vi "ScoreValidate.vi"(4 "Score":T2={"GUID"=0, "Score Mode Selector"=0, "Round Number"=0, "Full Score Entry"={"Elements"=[{"Name"="CO2 Balls Touching/Within Reservoir Model", "Value"="-1"}, {"Name"="Money Ball Touching/Within Reservoir Model", "Value"="-1"}, {"Name"="3+ Red/White Citizens in Pink Grid Area", "Value"="-1"}, {"Name"="# Upright Levee Blocks touching ONLY GREEN shores", "Value"="-1"}, {"Name"="# Upright Levee Blocks Touching any RED shore", "Value"="-1"}, {"Name"="Levee Test was Performed", "Value"="-1"}, {"Name"="Levee Test Wheel Blocked by NonLevee", "Value"="-1"}, {"Name"="Flood Barrier in Up Position", "Value"="-1"}, {"Name"="Both Yellow Arrows Aligned", "Value"="-1"}, {"Name"="Team Robot Touching Only Yellow Grid Area", "Value"="-1"}, {"Name"="Both Insulation Touching Green Grid Area", "Value"="-1"}, {"Name"="Bicycle Touching Green Grid Area", "Value"="-1"}, {"Name"="Computer Touching Green Grid Area", "Value"="-1"}, {"Name"="House in Up Position", "Value"="-1"}, {"Name"="House Window Showing Black", "Value"="-1"}, {"Name"="House Window All The Way Open", "Value"="-1"}, {"Name"="3+ Black/White Scientists Touching Research Area", "Value"="-1"}, {"Name"="Money Ball Touching/Within Research Area Model", "Value"="-1"}, {"Name"="Polar Bear Touching/Within Research Area Model", "Value"="-1"}, {"Name"="Polar Bear Orientation (Sleeping/Upright)", "Value"="-1"}, {"Name"="Ice Core Pulled From Its Hole", "Value"="-1"}, {"Name"="Ice Buoy Upright and Within/Touching Research Area Model", "Value"="-1"}, {"Name"="Drilling Machine Touching/Within Research Area Model", "Value"="-1"}, {"Name"="Drill Assembly Completely Vertical", "Value"="-1"}, {"Name"="Team Robot Touching/Within Research Area Model", "Value"="-1"}, {"Name"="3+ Blue/Gray Leaders Touching Green Mountain/City Area", "Value"="-1"}, {"Name"="Ice Core in Base Area", "Value"="-1"}, {"Name"="Snowmobile Touching/Within Research Area Model", "Value"="-1"}], "Score"=0.0}} {"Score Mode Selector" items=["Automatic", "Manual"]}, 5 "Scores":T1 {"Score"."Score Mode Selector" items=["Automatic", "Manual"]}) -> (0 "Errors":string, 1 "Index":i32, 2 "Scores Out":T1 {"Score"."Score Mode Selector" items=["Automatic", "Manual"]})   [LabVIEW 2013]
uses:
  Full Score Entry.ctl
  ScoreEntry.ctl
  ScoreList.ctl
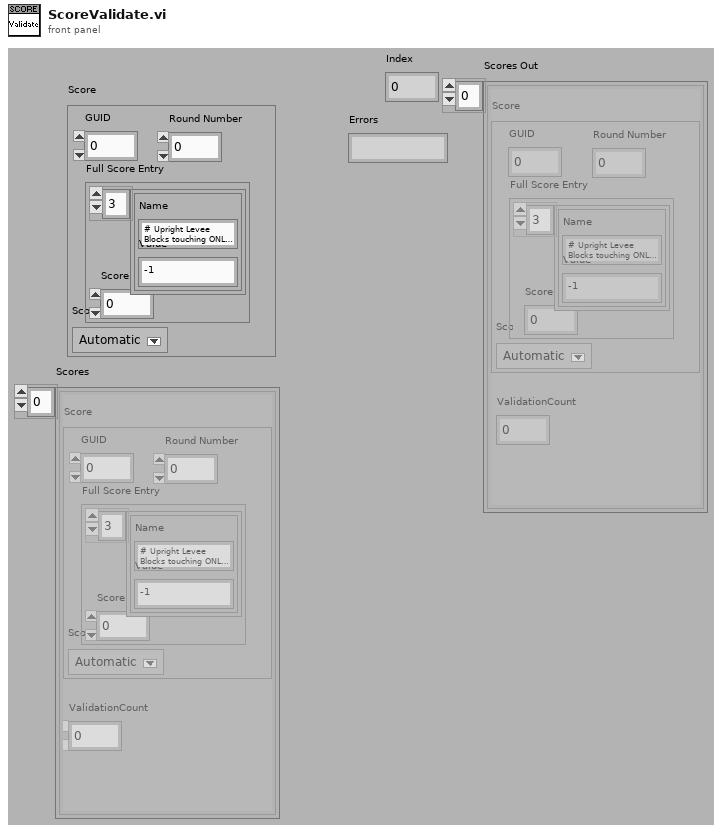
[diagram p1: front panel]
types:
  T1 = typedef "ScoreList.ctl" = cluster{"ValidationCount":u16, "Score":T2}[]
  T2 = typedef "Full Score Entry.ctl" = cluster{"GUID":u16, "Score Mode Selector":u16, "Round Number":u16, "Full Score Entry":T3}
  T3 = typedef "ScoreEntry.ctl" = cluster{"Elements":cluster{"Name":string, "Value":string}[], "Score":dbl}
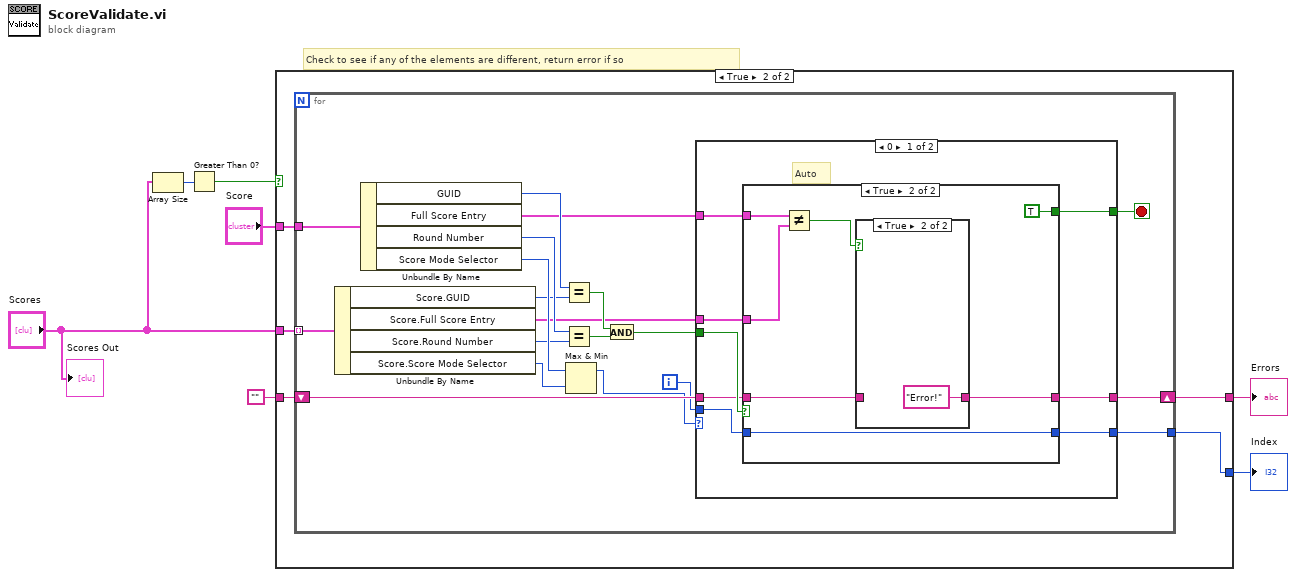
[diagram p0: block diagram]
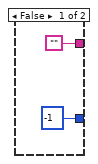
[diagram p2: hidden frame]
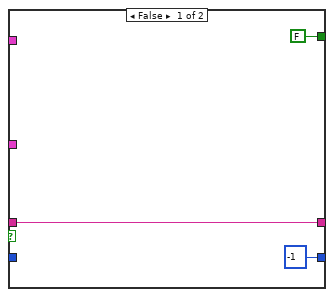
[diagram p3: hidden frame]
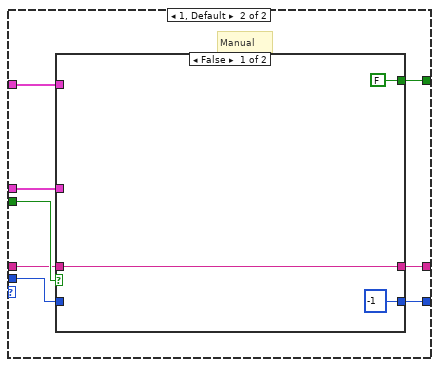
[diagram p5: hidden frame]
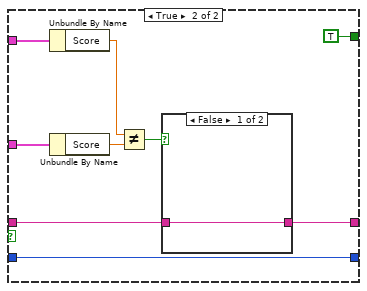
[diagram p6: hidden frame]
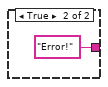
[diagram p7: hidden frame]
diagram:
  # "Check to see if any of the elements are different, return error if so"
  n1 = Array Size(array="Scores") -> (size(s)=w4:i32)
  n2 = Greater Than 0?(x=w4) -> (x > 0?=w3:bool)
  n3 = case shown="True" w3 {
    tunnel: "Score" -> [_ w14]
    tunnel: "" -> [_ w13]
    tunnel: ["" w12] -> w6
    tunnel: [-1 w11] -> w5
    tunnel: "Scores" -> [_ w10]
    frame False {
    }
    frame True {
      n4 = for {
        tunnel: w14 -> [w33]
        tunnel: w10 -> [w19] mode=indexing
        shift-right: [w25] -> w12
        shift-left: w13 -> [w26]
        tunnel: [w21] -> w11
        i -> [w22]
        stop <- w20 stop-if-true
        n5 = Unbundle By Name(w19) -> ("Score.GUID"=w18:u16, "Score.Full Score Entry"=w17:T3, "Score.Round Number"=w16:u16, "Score.Score Mode Selector"=w15:u16)
        n6 = Unbundle By Name(w33) -> ("GUID"=w32:u16, "Full Score Entry"=w27:T3, "Round Number"=w31:u16, "Score Mode Selector"=w24:u16)
        n7 = Equal?(x=w32, y=w18) -> (x = y?=w29:bool)
        n8 = Equal?(x=w31, y=w16) -> (x = y?=w30:bool)
        n9 = Max & Min(x=w24, y=w15) -> (max(x,y)=w23:u16)  [unwired: 1 out]
        n10 = And(x=w29, y=w30) -> (x .and. y?=w28:bool)
        n11 = case shown="0" w23 {
          tunnel: w28 -> [w41 w61]
          tunnel: w27 -> [w40 w60]
          tunnel: w17 -> [w39 w59]
          tunnel: w26 -> [w38 w58]
          tunnel: [w37 w57] -> w25
          tunnel: w22 -> [w36 w56]
          tunnel: [w35 w55] -> w21
          tunnel: [w34 w54] -> w20
          frame 0 {
            # "Auto"
            n12 = case shown="True" w41 {
              tunnel: w40 -> [_ w50]
              tunnel: w39 -> [_ w51]
              tunnel: w38 -> [w44 w48]
              tunnel: [w44 w47] -> w37
              tunnel: w36 -> [_ w46]
              tunnel: [-1 w46] -> w35
              tunnel: [FALSE TRUE] -> w34
              frame False {
              }
              frame True {
                n13 = Not Equal?(x=w50, y=w51) -> (x != y?=w49:bool)
                n14 = case shown="True" w49 {
                  tunnel: w48 -> [w52 _]
                  tunnel: [w52 "Error!"] -> w47
                  frame False {
                  }
                  frame True {
                  }
                }
              }
            }
          }
          frame 1, Default {
            # "Manual"
            n15 = case shown="False" w61 {
              tunnel: w60 -> [_ w69]
              tunnel: w59 -> [_ w70]
              tunnel: w58 -> [w64 w72]
              tunnel: [w64 w71] -> w57
              tunnel: w56 -> [_ w66]
              tunnel: [-1 w66] -> w55
              tunnel: [FALSE TRUE] -> w54
              frame False {
              }
              frame True {
                n16 = Unbundle By Name(w69) -> ("Score"=w68:dbl)
                n17 = Unbundle By Name(w70) -> ("Score"=w67:dbl)
                n18 = Not Equal?(x=w68, y=w67) -> (x != y?=w73:bool)
                n19 = case shown="False" w73 {
                  tunnel: w72 -> [w74 _]
                  tunnel: [w74 "Error!"] -> w71
                  frame False {
                  }
                  frame True {
                  }
                }
              }
            }
          }
        }
      }
    }
  }
  "Errors" <- w6
  "Index" <- w5
  "Scores Out" <- "Scores"
